vi "Test config class.vi"() -> ()   [LabVIEW 2026]
uses:
  Classes/Config/Config.lvclass
  Classes/Config/Get Parameter Value - Array of Strings.vi
  Classes/Config/Get Parameter Value - Array of Doubles.vi
  Classes/Config/Get Parameter Value - Array of Integers.vi
  Classes/Config/Get Parameter Value - Array of Booleans.vi
  Classes/Config/Get Current Parameter Value - Array of Strings.vi
  Classes/Config/Get Current Parameter Value - Array of Doubles.vi
  Classes/Config/Get Current Parameter Value - Array of Integers.vi
  Classes/Config/Get Current Parameter Value - Array of Booleans.vi
panel:
  out "Log information":string
  in  "Path":path=path "C:/LabVIEW Code/TALOS/talos/Test Stuff/test_config.ini"
  in  "Load config":bool
  in  "Select mode":bool=TRUE
  in  "Test config":string
  out "Current Config":string
  in  "Clear errors":bool
  out "error out":errorcluster[](array[cluster])
  in  "Data type":T1(ring)
  out "output selector":T2(tab)
  out "String value":string
  in  "Default string":string caption="Default value"
  out "Double value":dbl
  in  "Default double":dbl caption="Default value"
  out "Integer value":i32 caption="Double value"
  in  "Default integer":i32 caption="Default value"
  out "Boolean value":bool caption="Double value"
  in  "Default bool":bool caption="Default value"
  out "Array of strings":string[](array[string])
  in  "Default Array[str]":string[](array[string]) caption="Default value"
  out "Array of doubles":dbl[](array[numeric]) caption="Double value"
  in  "Default Array[dbl]":dbl[](array[numeric]) caption="Default value"
  out "Array of integers":i32[](array[numeric]) caption="Double value"
  in  "Default Array[int]":i32[](array[numeric]) caption="Default value"
  out "Array of booleans":bool[](array[boolean]) caption="Double value"
  in  "Default Array[bool]":bool[](array[boolean]) caption="Default value"
  in  "Parameter name":string
  in  "Get current param":bool
  in  "Set config":bool
  in  "Get parameter":bool
  in  "Config name":string(combo)
  in  "EXIT":bool
  out "loaded config file":path
  # "Use test config\nspace"
  # "Load specific\nfile"
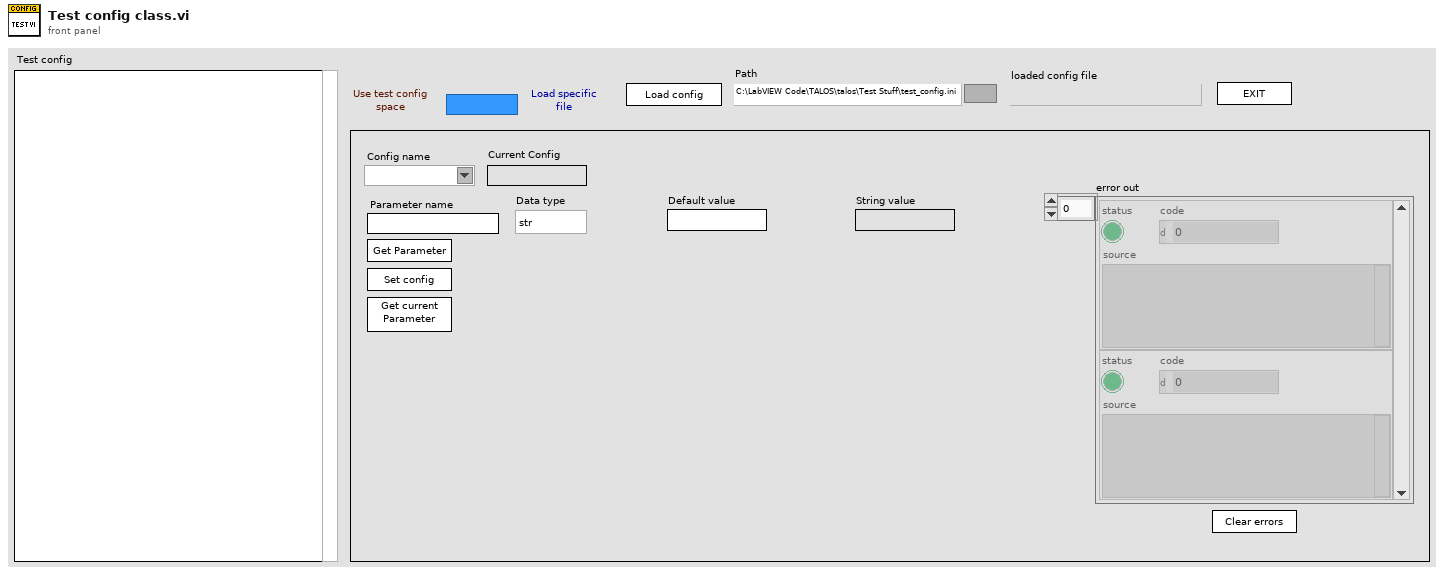
[diagram p1: front panel]
types:
  T1 = enum16{"str", "dbl", "int", "bool", "Array[str]", "Array[dbl]", "Array[int]", "Array[bool]"}
  T2 = enum32{"str", "dbl", "int", "bool", "Array[str]", "Array[dbl]", "Array[int]", "Array[bool]"}
  T3 = enum8{"Enabled", "Disabled", "Disabled and Grayed Out"}
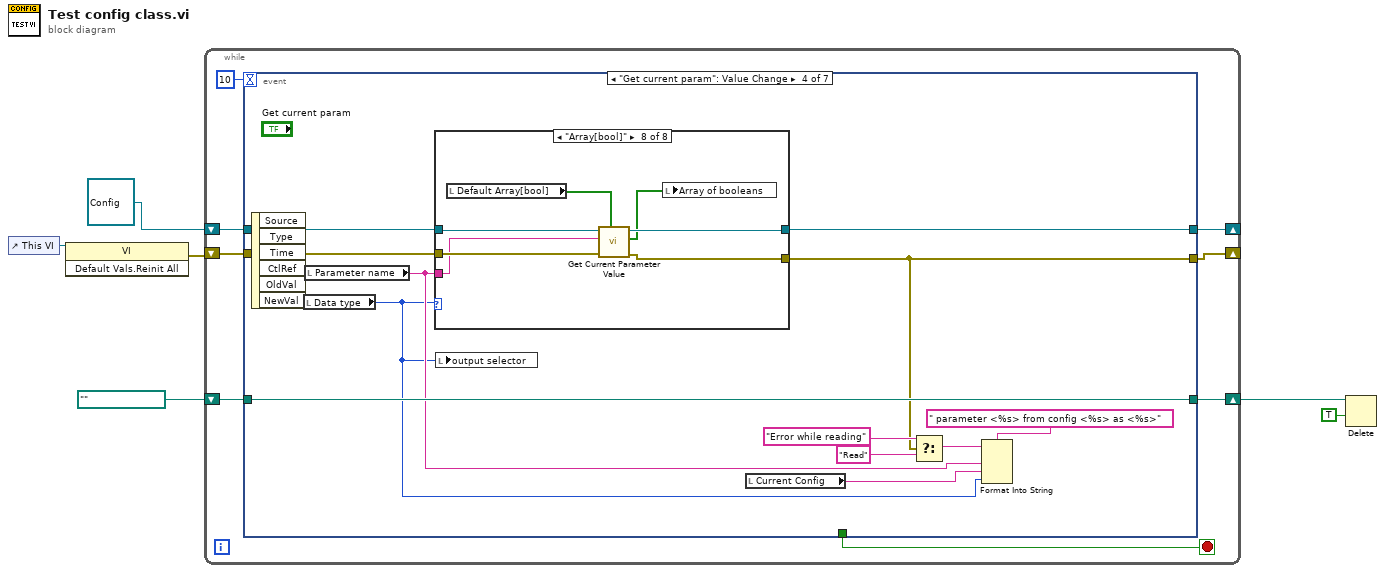
[diagram p0: block diagram]
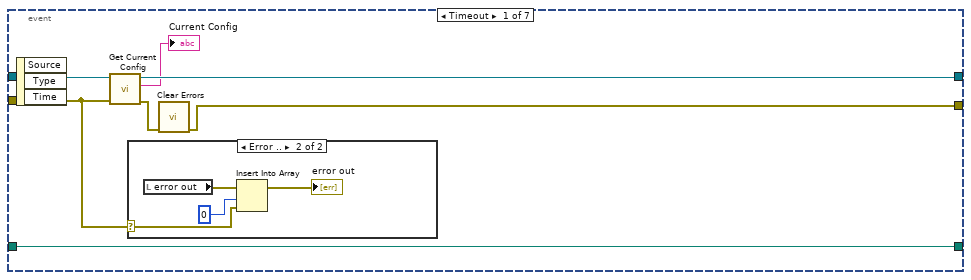
[diagram p2: hidden frame]
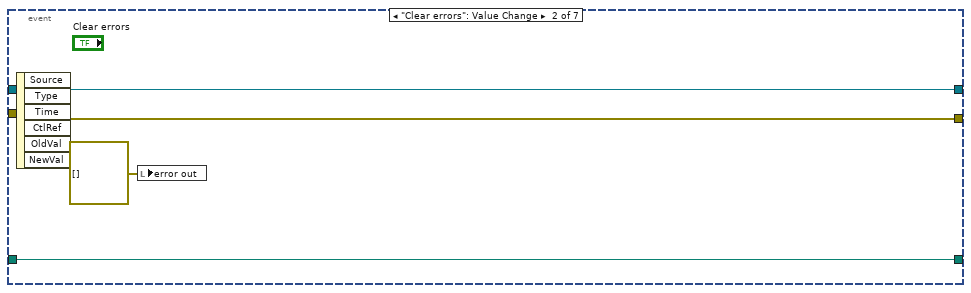
[diagram p4: hidden frame]
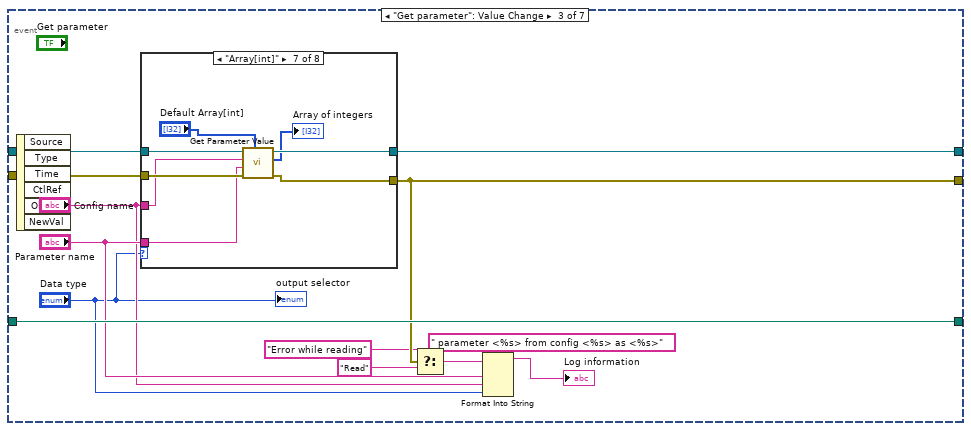
[diagram p5: hidden frame]
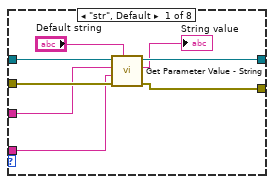
[diagram p6: hidden frame]
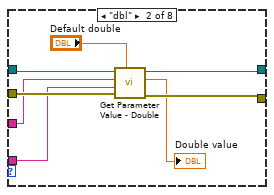
[diagram p7: hidden frame]
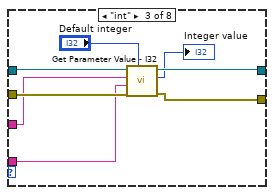
[diagram p8: hidden frame]
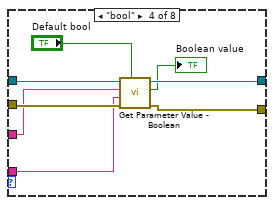
[diagram p9: hidden frame]
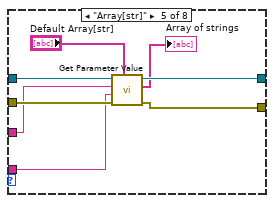
[diagram p10: hidden frame]
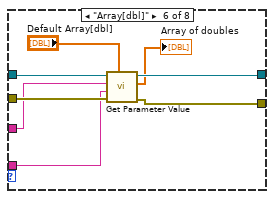
[diagram p11: hidden frame]
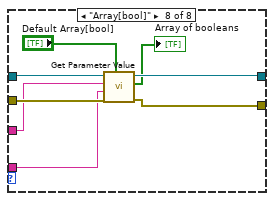
[diagram p12: hidden frame]
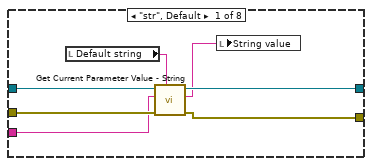
[diagram p13: hidden frame]
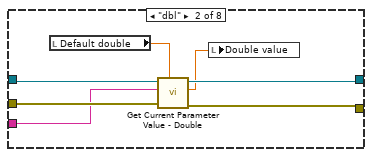
[diagram p14: hidden frame]
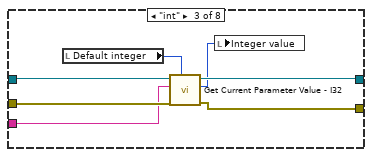
[diagram p15: hidden frame]
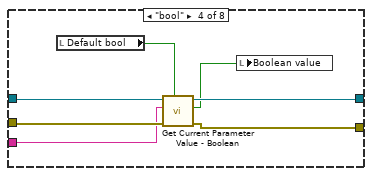
[diagram p16: hidden frame]
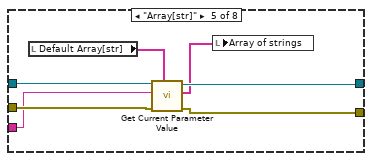
[diagram p17: hidden frame]
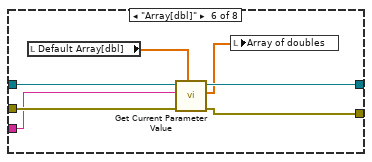
[diagram p18: hidden frame]
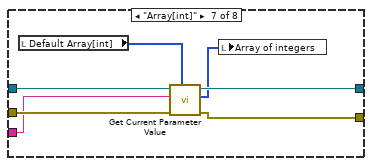
[diagram p19: hidden frame]
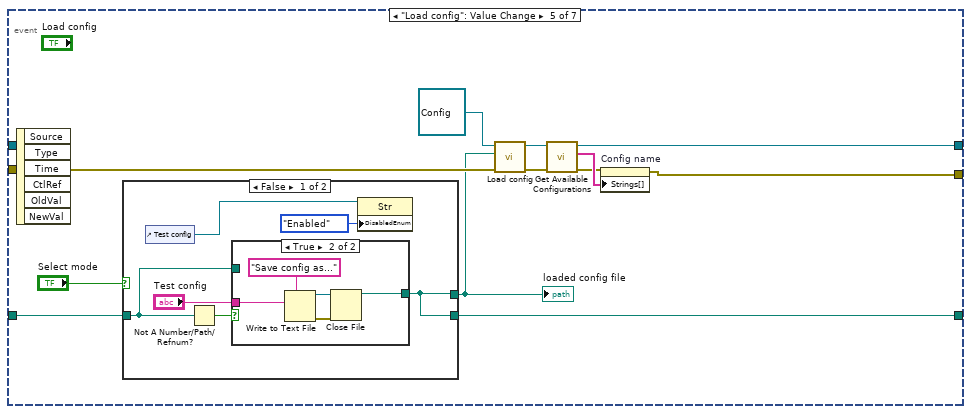
[diagram p20: hidden frame]
diagram:
  n1 = control-ref of="This VI"() -> (w6:refnum<vi>)
  n2 = invoke class="VI" method="Default Vals.Reinit All"(reference=w6) -> (error out=w4:errorcluster)  [unwired: 2 in, 2 out]
  n3 = while {
    shift-right: [w12] -> _
    shift-left: refnum<class "Config.lvclass"> refnum ("Config out") -> [w13]
    shift-right: [w9] -> _
    shift-left: w4 -> [w11]
    shift-right: [w7] -> w2
    shift-left: path "" ("file (use dialog)") -> [w8]
    stop <- w14 stop-if-true
    n4 = event shown="[3] \"Get current param\": Value Change" {
      selector: _ -> [_ _ _ _ _ _ _]
      dyn-events: _ -> [_ _ _ _ _ _ _]
      timeout: 10 -> [_ _ _ _ _ _ _]
      tunnel: [_ _ _ _ _ _ "EXIT"] -> w14
      tunnel: w13 -> [w20 w28 w42 w118 _ w216 w219]
      tunnel: [w17 w28 w40 w116 w181 w214 w219] -> w12
      tunnel: w11 -> [w19 w29 w41 w117 w179 w215 w218]
      tunnel: [w21 w29 w33 w110 w180 w213 w218] -> w9
      tunnel: w8 -> [w15 w26 w39 w115 w177 w212 w217]
      tunnel: [w15 w26 w39 w115 w176 w212 w217] -> w7
      event Timeout {
        n5 = event-data() -> ()  [unwired: 1 in, 3 out]
        n6 = call-dynamic "Get Current Config.vi"("error in (no error)"=w19, "Config in"=w20) -> ("error out"=w18:errorcluster, "Current Config"=→"Current Config":string, "Config out"=w17:refnum<class "Config.lvclass">)  [unwired: 7 in]
        n7 = case shown="Error .." w19 {
          selector: w19 -> [_ w24]
          frame No Error {
          }
          frame Error {
            n8 = local read "error out"() -> (w25:errorcluster[])
            n9 = Insert Into Array(array=w25, index=0, new element=w24) -> (→"error out":errorcluster[])
          }
        }
        n10 = call <vilib>:"Clear Errors.vi"("error in (no error)"=w18) -> ("error out"=w21:errorcluster)  [unwired: 5 in, 1 out]
      }
      event "Clear errors": Value Change {
        n11 = event-data() -> ()  [unwired: 1 in, 6 out]
        n12 = local write "error out"(errorcluster[] [] ("error out")) -> ()
      }
      event "Get parameter": Value Change {
        n13 = event-data() -> ()  [unwired: 1 in, 6 out]
        n14 = case shown="\"Array[int]\"" "Data type" {
          tunnel: w42 -> [w49 w58 w66 w74 w82 w90 w98 w106]
          tunnel: w41 -> [w48 w57 w65 w71 w79 w89 w95 w105]
          tunnel: [w47 w56 w63 w72 w80 w87 w96 w101] -> w33
          tunnel: [w46 w55 w64 w73 w81 w88 w97 w100] -> w40
          tunnel: "Config name" -> [w44 w53 w59 w70 w78 w86 w94 w104]
          tunnel: "Parameter name" -> [w43 w52 w60 w69 w77 w85 w93 w103]
          frame "str", Default {
            n15 = call "Get Parameter Value - String.vi"("Default value"="Default string", "error in (no error)"=w48, "Parameter name"=w43, "Config name"=w44, "Config in"=w49) -> ("error out"=w47:errorcluster, "Value"=→"String value":string, "Config out"=w46:refnum<class "Config.lvclass">)  [unwired: 4 in]
          }
          frame "dbl" {
            n16 = call "Get Parameter Value - Double.vi"("Default value"="Default double", "error in (no error)"=w57, "Parameter name"=w52, "Config name"=w53, "Config in"=w58) -> ("error out"=w56:errorcluster, "Value"=→"Double value":dbl, "Config out"=w55:refnum<class "Config.lvclass">)  [unwired: 4 in]
          }
          frame "int" {
            n17 = call "Get Parameter Value - I32.vi"("Default value"="Default integer", "error in (no error)"=w65, "Parameter name"=w60, "Config name"=w59, "Config in"=w66) -> ("error out"=w63:errorcluster, "Value"=→"Integer value":i32, "Config out"=w64:refnum<class "Config.lvclass">)  [unwired: 4 in]
          }
          frame "bool" {
            n18 = call "Get Parameter Value - Boolean.vi"("Default value"="Default bool", "error in (no error)"=w71, "Parameter name"=w69, "Config name"=w70, "Config in"=w74) -> ("error out"=w72:errorcluster, "Value"=→"Boolean value":bool, "Config out"=w73:refnum<class "Config.lvclass">)  [unwired: 4 in]
          }
          frame "Array[str]" {
            n19 = call-poly "Get Parameter Value.vi"("Default value"="Default Array[str]", "error in (no error)"=w79, "Parameter name"=w77, "Config name"=w78, "Config in"=w82) -> ("error out"=w80:errorcluster, "Value"=→"Array of strings":string[], "Config out"=w81:refnum<class "Config.lvclass">)  [unwired: 4 in]
          }
          frame "Array[dbl]" {
            n20 = call-poly "Get Parameter Value.vi"("Default value"="Default Array[dbl]", "error in (no error)"=w89, "Parameter name"=w85, "Config name"=w86, "Config in"=w90) -> ("error out"=w87:errorcluster, "Value"=→"Array of doubles":dbl[], "Config out"=w88:refnum<class "Config.lvclass">)  [unwired: 4 in]
          }
          frame "Array[int]" {
            n21 = call-poly "Get Parameter Value.vi"("Default value"="Default Array[int]", "error in (no error)"=w95, "Parameter name"=w93, "Config name"=w94, "Config in"=w98) -> ("error out"=w96:errorcluster, "Value"=→"Array of integers":i32[], "Config out"=w97:refnum<class "Config.lvclass">)  [unwired: 4 in]
          }
          frame "Array[bool]" {
            n22 = call-poly "Get Parameter Value.vi"("Default value"="Default Array[bool]", "error in (no error)"=w105, "Parameter name"=w103, "Config name"=w104, "Config in"=w106) -> ("error out"=w101:errorcluster, "Value"=→"Array of booleans":bool[], "Config out"=w100:refnum<class "Config.lvclass">)  [unwired: 4 in]
          }
        }
        n23 = Select(t="Error while reading" ("Parameter name"), s=w33, f="Read" ("Parameter name")) -> (s? t:f=w30:string)
        n24 = Format Into String(format string=" parameter <%s> from config <%s> as <%s>", initial string=w30, "Parameter name", "Config name", "Data type") -> (resulting string=→"Log information":string)  [unwired: 1 in, 1 out]
        "output selector" <- "Data type"
      }
      event "Get current param": Value Change {
        n25 = event-data() -> ()  [unwired: 1 in, 6 out]
        n26 = local read "Data type"() -> (w107:T1)
        n27 = local read "Parameter name"() -> (w109:string)
        n28 = case shown="\"Array[bool]\"" w107 {
          tunnel: w118 -> [w125 w132 w139 w146 w153 w160 w167 w174]
          tunnel: w117 -> [w124 w131 w138 w143 w152 w159 w165 w173]
          tunnel: [w123 w130 w136 w144 w150 w157 w164 w171] -> w110
          tunnel: [w122 w129 w137 w145 w151 w158 w166 w172] -> w116
          tunnel: w109 -> [w121 w128 w135 w142 w149 w156 w163 w170]
          frame "str", Default {
            n29 = local read "Default string"() -> (w119:string)
            n30 = call "Get Current Parameter Value - String.vi"("Default value"=w119, "error in (no error)"=w124, "Parameter name"=w121, "Config in"=w125) -> ("error out"=w123:errorcluster, "Value"=w120:string, "Config out"=w122:refnum<class "Config.lvclass">)  [unwired: 5 in]
            n31 = local write "String value"(w120) -> ()
          }
          frame "dbl" {
            n32 = local read "Default double"() -> (w126:dbl)
            n33 = call "Get Current Parameter Value - Double.vi"("Default value"=w126, "error in (no error)"=w131, "Parameter name"=w128, "Config in"=w132) -> ("error out"=w130:errorcluster, "Value"=w127:dbl, "Config out"=w129:refnum<class "Config.lvclass">)  [unwired: 5 in]
            n34 = local write "Double value"(w127) -> ()
          }
          frame "int" {
            n35 = local read "Default integer"() -> (w133:i32)
            n36 = call "Get Current Parameter Value - I32.vi"("Default value"=w133, "error in (no error)"=w138, "Parameter name"=w135, "Config in"=w139) -> ("error out"=w136:errorcluster, "Value"=w134:i32, "Config out"=w137:refnum<class "Config.lvclass">)  [unwired: 5 in]
            n37 = local write "Integer value"(w134) -> ()
          }
          frame "bool" {
            n38 = local read "Default bool"() -> (w140:bool)
            n39 = call "Get Current Parameter Value - Boolean.vi"("Default value"=w140, "error in (no error)"=w143, "Parameter name"=w142, "Config in"=w146) -> ("error out"=w144:errorcluster, "Value"=w141:bool, "Config out"=w145:refnum<class "Config.lvclass">)  [unwired: 5 in]
            n40 = local write "Boolean value"(w141) -> ()
          }
          frame "Array[str]" {
            n41 = local read "Default Array[str]"() -> (w148:string[])
            n42 = call-poly "Get Current Parameter Value.vi"("Default value"=w148, "error in (no error)"=w152, "Parameter name"=w149, "Config in"=w153) -> ("error out"=w150:errorcluster, "Value"=w147:string[], "Config out"=w151:refnum<class "Config.lvclass">)  [unwired: 5 in]
            n43 = local write "Array of strings"(w147) -> ()
          }
          frame "Array[dbl]" {
            n44 = local read "Default Array[dbl]"() -> (w155:dbl[])
            n45 = call-poly "Get Current Parameter Value.vi"("Default value"=w155, "error in (no error)"=w159, "Parameter name"=w156, "Config in"=w160) -> ("error out"=w157:errorcluster, "Value"=w154:dbl[], "Config out"=w158:refnum<class "Config.lvclass">)  [unwired: 5 in]
            n46 = local write "Array of doubles"(w154) -> ()
          }
          frame "Array[int]" {
            n47 = local read "Default Array[int]"() -> (w162:i32[])
            n48 = call-poly "Get Current Parameter Value.vi"("Default value"=w162, "error in (no error)"=w165, "Parameter name"=w163, "Config in"=w167) -> ("error out"=w164:errorcluster, "Value"=w161:i32[], "Config out"=w166:refnum<class "Config.lvclass">)  [unwired: 5 in]
            n49 = local write "Array of integers"(w161) -> ()
          }
          frame "Array[bool]" {
            n50 = local read "Default Array[bool]"() -> (w169:bool[])
            n51 = call-poly "Get Current Parameter Value.vi"("Default value"=w169, "error in (no error)"=w173, "Parameter name"=w170, "Config in"=w174) -> ("error out"=w171:errorcluster, "Value"=w168:bool[], "Config out"=w172:refnum<class "Config.lvclass">)  [unwired: 5 in]
            n52 = local write "Array of booleans"(w168) -> ()
          }
        }
        n53 = local write "output selector"(w107) -> ()
        n54 = local read "Current Config"() -> (w108:string)
        n55 = Select(t="Error while reading" ("Parameter name"), s=w110, f="Read" ("Parameter name")) -> (s? t:f=w113:string)
        n56 = Format Into String(format string=" parameter <%s> from config <%s> as <%s>", initial string=w113, w109, w108, w107) -> ()  [unwired: 1 in, 2 out]
      }
      event "Load config": Value Change {
        n57 = event-data() -> ()  [unwired: 1 in, 6 out]
        n58 = case shown="False" "Select mode" {
          tunnel: [w190 w206] -> w175
          tunnel: w177 -> [w189 w210]
          tunnel: [w190 w210] -> w176
          frame False {
            n59 = control-ref of="Test config"() -> (w188:refnum<vi>)
            n60 = Not A Number/Path/Refnum?(number/path/refnum=w189) -> (NaN/Path/Refnum?=w191:bool)
            n61 = case shown="True" w191 {
              tunnel: "Test config" -> [w194 w202]
              tunnel: [w195 w198] -> w190
              tunnel: w189 -> [w193 _]
              frame False {
                n62 = Write to Text File(file (use dialog)=w193, text=w194) -> (refnum out=w197:refnum<file>, error out=w196:errorcluster)  [unwired: 2 in, 1 out]
                n63 = Close File(refnum=w197, error in=w196) -> (path=w195:path)  [unwired: 1 out]
              }
              frame True {
                n64 = Write to Text File(prompt (Choose or enter file path)="Save config as...", text=w202) -> (refnum out=w200:refnum<file>, error out=w201:errorcluster)  [unwired: 2 in, 1 out]
                n65 = Close File(refnum=w200, error in=w201) -> (path=w198:path)  [unwired: 1 out]
              }
            }
            n66 = property on="Property Node" class="Str"(reference=w188, "DisabledEnum"=T3."Enabled" ("Disabled")) -> ()  [unwired: 1 in, 2 out]
          }
          frame True {
            n67 = control-ref of="Test config"() -> (w203:refnum<vi>)
            n68 = Read from Text File(file (use dialog)="Path") -> (refnum out=w207:refnum<file>, text=w205:string, error out=w208:errorcluster)  [unwired: 3 in, 1 out]
            n69 = Close File(refnum=w207, error in=w208) -> (path=w206:path)  [unwired: 1 out]
            n70 = property on="Property Node" class="Str"(reference=w203, "DisabledEnum"=T3."Disabled" ("Disabled"), "Value"=w205) -> ()  [unwired: 1 in, 2 out]
          }
        }
        "loaded config file" <- w175
        n71 = call "Load config.vi"("error in"=w179, "config file path"=w175, "Config in"=refnum<class "Config.lvclass"> refnum) -> ("error out"=w184:errorcluster, "Config out"=w183:refnum<class "Config.lvclass">)  [unwired: 7 in]
        n72 = call-dynamic "Get Available Configurations.vi"("error in (no error)"=w184, "Config in"=w183) -> ("error out"=w185:errorcluster, "Configuration names"=w186:string[], "Config out"=w181:refnum<class "Config.lvclass">)  [unwired: 7 in]
        n73 = property on="Config name" class="CmbBox"(error in=w185, "Strings[]"=w186) -> (error out=w180:errorcluster)  [unwired: 1 in, 1 out]
      }
      event "Set config": Value Change {
        n74 = event-data() -> ()  [unwired: 1 in, 6 out]
        n75 = local read "Config name"() -> (w211:string)
        n76 = call-dynamic "Set Configuration.vi"("error in (no error)"=w215, "Config name"=w211, "Config in"=w216) -> ("error out"=w213:errorcluster, "Config out"=w214:refnum<class "Config.lvclass">)  [unwired: 6 in, 1 out]
      }
      event "EXIT": Value Change {
        n77 = event-data() -> ()  [unwired: 1 in, 6 out]
      }
    }
  }
  n78 = Delete(path (use dialog)=w2, confirm (F)=TRUE) -> ()  [unwired: 3 in, 3 out]
